vi "Integration Query.vi"(8 "error in (no error)":errorcluster, 11 "Yokogawa WT2X0 in":refnum<class "Yokogawa WT2X0.lvclass">) -> (0 "error out":errorcluster, 1 "Integration State":T1, 3 "Yokogawa WT2X0 out":refnum<class "Yokogawa WT2X0.lvclass">)   [LabVIEW 2013]
uses:
  Yokogawa WT2X0.lvclass
  <instrlib>/Yokogawa WT200 Series/Yokogawa WT200 Series.lvlib
  Universal Power Meter class/Integration State.ctl
  Universal Power Meter class/Universal Power Meter.lvclass
panel:
  out "output string":string
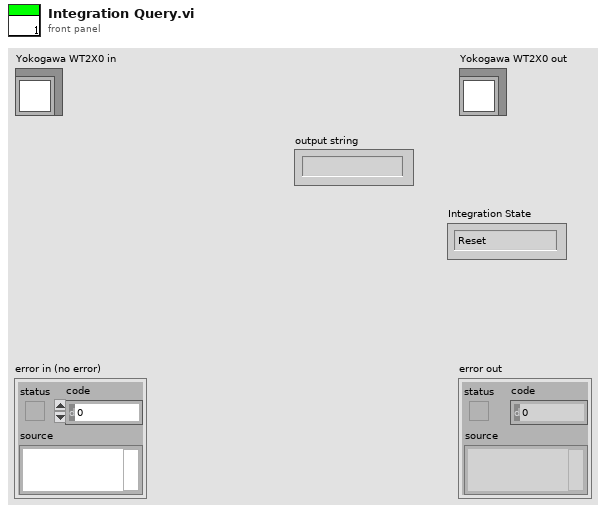
[diagram p1: front panel]
types:
  T1 = typedef "Universal Power Meter.lvlib/Universal Power Meter.lvclass/Integration State.ctl" = enum16{"Reset", "Stop", "Start"}
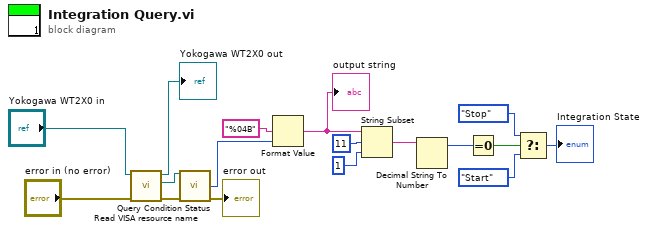
[diagram p0: block diagram]
diagram:
  n1 = call-dynamic "Read VISA resource name.vi"("error in (no error)"="error in (no error)", "Generic Instrument in"="Yokogawa WT2X0 in") -> ("error out"=w3:errorcluster, "VISA resource name"=w16:refnum<visa-resource-name>, "Generic Instrument out"=→"Yokogawa WT2X0 out":refnum<class "Yokogawa WT2X0.lvclass">)  [unwired: 7 in]
  n2 = call <instrlib>:"Query Condition Status.vi"("VISA resource name"=w16, "error in (no error)"=w3) -> ("Condition"=w11:i16, "error out"=→"error out":errorcluster)  [unwired: 11 in, 1 out]
  n3 = Format Value(format string="%04B", value (0)=w11) -> (output string=w13:string)  [unwired: 1 in]
  "output string" <- w13
  n4 = String Subset(string=w13, offset (0)=11, length (rest)=1 ("length (rest)")) -> (substring=w10:string)
  n5 = Decimal String To Number(string=w10) -> (offset past number=w9:i32)  [unwired: 2 in, 1 out]
  n6 = Equal To 0?(x=w9) -> (x = 0?=w8:bool)
  n7 = Select(t=Integration_State."Stop" ("Integration State"), s=w8, f=Integration_State."Start" ("Integration State")) -> (s? t:f=→"Integration State":T1)
